vi "device on off array to DB.vi"(0 "String in":refnum<vi>, 1 "ItemSyms 3":i32[](array[numeric]), 2 "Array":i32[](array[numeric]), 5 "user event in":refnum<user-event>, 7 "Array 2":bool[](array[boolean]), 9 "Stop Devices on Remove":bool=TRUE, 11 "error in (no error)":errorcluster, 12 "ItemNames":string[][](array[string]), 13 "Value":string) -> (4 "ItemSyms":i32[](array[numeric]), 6 "ItemSyms 2":i32[](array[numeric]))   [LabVIEW 2020]
uses:
  <userlib>/_OpenG.lib/array/array.llb/Search 1D Array (Boolean)__ogtk.vi
  <userlib>/_OpenG.lib/array/array.llb/Index 1D Array Elements (I32)__ogtk.vi
  <userlib>/_OpenG.lib/array/array.llb/Index 1D Array Elements (String)__ogtk.vi
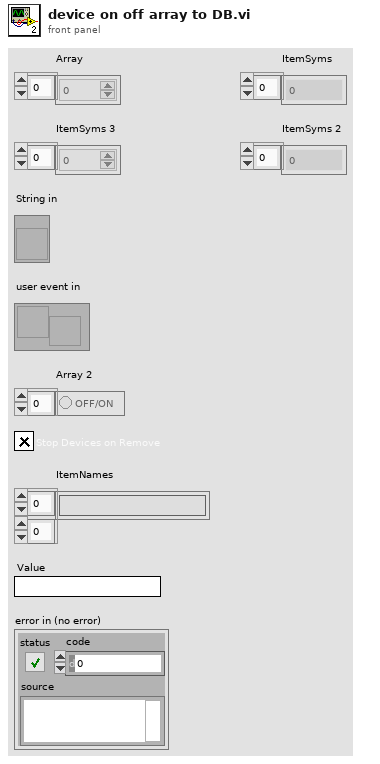
[diagram p1: front panel]
types:
  T1 = typedef "mysql_authentication.ctl" = cluster{"User":string, "Password":string, "Database":string}
  T2 = cluster{"Port":u16, "IP Address":string, "Authentication":T1}
  T3 = cluster{"Message":string, "Devices":string[], "stop devices":bool}
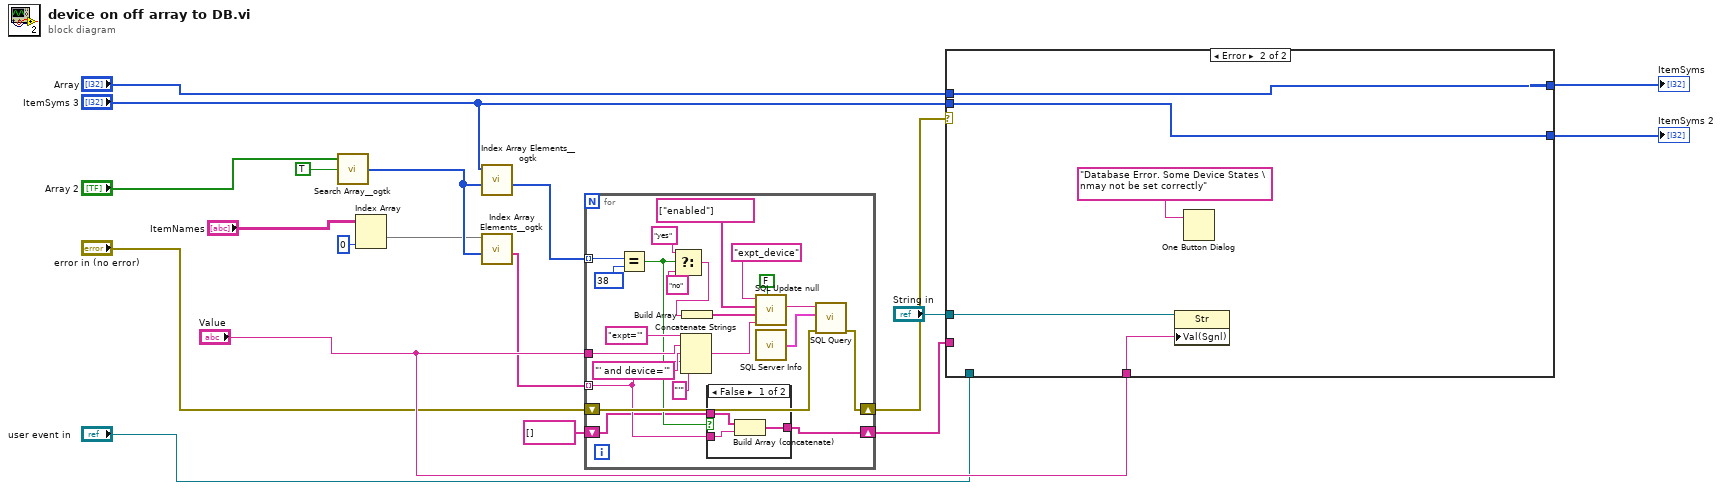
[diagram p0: block diagram]
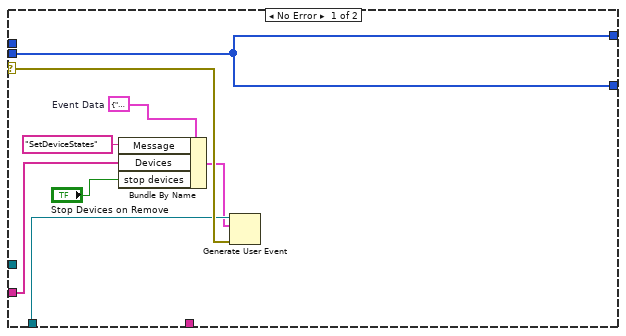
[diagram p2: hidden frame]
diagram:
  n1 = call-poly <userlib>:"Search Array__ogtk.vi"("Array"="Array 2", "Element Data"=TRUE ("element")) -> ("Indices of Elements"=w7:i32[])  [unwired: 7 in]
  n2 = Index Array(array="ItemNames", index (col)=0 ("disabled index (col)")) -> (element=w6:string[])  [unwired: 1 in]
  n3 = call-poly <userlib>:"Index Array Elements__ogtk.vi"("indices"=w7, "array"="ItemSyms 3") -> ("elements"=w8:i32[])  [unwired: 9 in]
  n4 = call-poly <userlib>:"Index Array Elements__ogtk.vi"("indices"=w7, "array"=w6) -> ("elements"=w9:string[])  [unwired: 9 in]
  n5 = for {
    tunnel: w8 -> [w36] mode=indexing
    tunnel: w9 -> [w22] mode=indexing
    tunnel: "Value" -> [w27]
    shift-right: [w24] -> w11
    shift-left: "error in (no error)" -> [w25]
    shift-right: [w21] -> w18
    shift-left: string[] [] -> [w20]
    n6 = Equal?(x=w36, y=38) -> (x = y?=w23:bool)
    n7 = Select(t="yes" ("Table"), s=w23, f="no" ("Table")) -> (s? t:f=w31:string)
    n8 = Concatenate Strings("expt='", w27, "' and device='" ("string"), w22, "'" ("string")) -> (w28:string)
    n9 = Build Array(w31) -> (w32:string[])
    n10 = case shown="False" w23 {
      tunnel: w22 -> [w44 _]
      tunnel: [w43 w45] -> w21
      tunnel: w20 -> [w42 w45]
      frame False {
        n11 = Build Array (concatenate)(w42, w44) -> (w43:string[])
      }
      frame True {
      }
    }
    n12 = call "SQL Update null.vi"("Use Empty String as Ignore? (T)"=FALSE, "Where clause"=w28, "Values"=w32, "Column Names"=string[] ["enabled"], "Table"="expt_device") -> ("Query String"=w39:string)  [unwired: 6 in]
    n13 = call "SQL Server Info.vi"() -> ("SQL Server Info"=w38:T2)
    n14 = call "SQL Query.vi"("error in (no error)"=w25, "SQL Server Info"=w38, "Query"=w39) -> ("error out"=w24:errorcluster)  [unwired: 7 in, 1 out]
  }
  n15 = case shown="Error" w11 {
    selector: w11 -> [w52 _]
    tunnel: "ItemSyms 3" -> [w53 w58]
    tunnel: [w53 w58] -> w13
    tunnel: [w53 w57] -> w14
    tunnel: "Array" -> [_ w57]
    tunnel: "user event in" -> [w49 _]
    tunnel: w18 -> [w50 _]
    tunnel: "Value" -> [_ w55]
    tunnel: "String in" -> [_ w54]
    frame No Error {
      w47 = T3 {"Message"="", "Devices"=[], "stop devices"=FALSE}  # Event Data
      n16 = Bundle By Name(cluster=w47, "Message"="SetDeviceStates" ("event data"), "Devices"=w50, "stop devices"="Stop Devices on Remove") -> (w48:T3)
      n17 = Generate User Event(user event=w49, event data cluster=w48, error in=w52) -> ()  [unwired: 1 in, 2 out]
    }
    frame Error {
      n18 = property on="Property Node" class="Str"(reference=w54, "Val(Sgnl)"=w55) -> ()  [unwired: 1 in, 2 out]
      n19 = One Button Dialog(message="Database Error. Some Device States \nmay not be set correctly") -> ()  [unwired: 1 in, 1 out]
    }
  }
  "ItemSyms" <- w14
  "ItemSyms 2" <- w13
